vi "Pre Launch Init.vi"(11 "Measurement Timer in":refnum<class "Measurement Timer.lvclass">) -> (0 "error out":errorcluster, 3 "Measurement Timer out":refnum<class "Measurement Timer.lvclass">)   [LabVIEW 2015, in "Measurement Timer.lvclass"]
doc: "(<B>Filename</B>: Actor Framework.lvlib:Actor.lvclass:Pre Launch Init.vi)\n\nDefines behavior that occurs after the Launch Actor method is invoked but before the actor's Actor Core method begins running.\n\nThe Pre Launch Init method is guaranteed to finish before the Launch Actor method returns to its caller and before the actor itself receives any messages. Any references that the Pre Launch Init method obtains are guaranteed to have the same lifetime as the actor itself. Any errors that the Pre Launch Init method returns will abort the launch.\n\nBy default, this method does nothing. A descendant class may override it to define behavior."
uses:
  Measurement Timer.lvclass
  Measurement Timer.lvclass/Measurement Timer.ctl
  Mag Lab Measurement/Mag Lab Measurement.lvclass
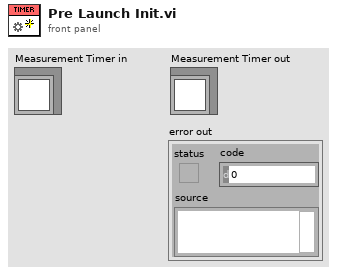
[diagram p1: front panel]
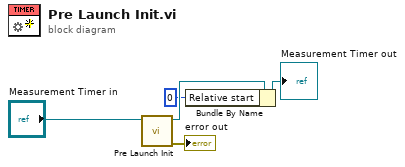
[diagram p0: block diagram]
diagram:
  n1 = call-parent "Pre Launch Init.vi"("Mag Lab Measurement in"="Measurement Timer in") -> ("error out"=→"error out":errorcluster, "Mag Lab Measurement out"=w4:refnum<class "Measurement Timer.lvclass">)  [unwired: 9 in]
  n2 = Bundle By Name(cluster=w4, "Relative start"=u64 0) -> (→"Measurement Timer out":refnum<class "Measurement Timer.lvclass">)
